vi "Error.vi"(8 "error in (no error)":errorcluster, 11 "Data":variant) -> (0 "error out":errorcluster)   [LabVIEW 2014, in "Testing UI 1.lvlib"]
doc: "This subVI enqueues the named action in to the communications queue along with the input data."
uses:
  Testing UI 1.lvlib
  Private Controls/Module Data.ctl
  Private Controls/Module Action.ctl
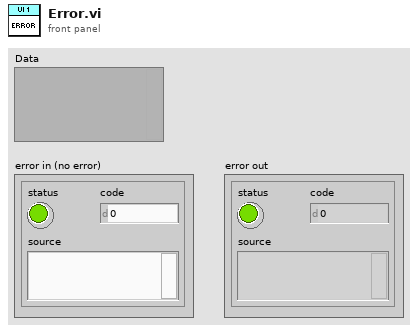
[diagram p1: front panel]
types:
  T1 = typedef "Testing UI 1.lvlib/Module Data.ctl" = cluster{"Data":variant, "Action":T2}
  T2 = typedef "Testing UI 1.lvlib/Module Action.ctl" = enum8{"Init", "Error", "Exit", "HideShow FP", "Send Control Vals", "New Message Line", "Update System Log", "Load APU Setup Data", "Update APU Name", "Set Testing Type", "Threshold ALERT", "Set Rapid OpenORClose", "Engine Start Val Change", "Fault Trip Run Updater", " ---------------UI 4 APIs ---------------", "UI 4 Engine Start Val Change", "UI 4 Fuel Pressure Reg Val Change", "U1 4 APU & ECU Control Val Change", "UI 4 Bleed Load Val Change", "UI4 Testing Controls Val Change", "UI4 Break Out Val Change", "UI4 Crash Log Val Change", "UI4 Log Data Val Change", "UI4 Sampes-Sec Val Change", "Update Run Count", "Config Interactive Ctrls"}
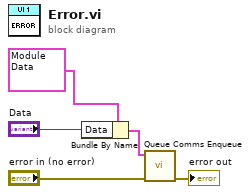
[diagram p0: block diagram]
diagram:
  n1 = Bundle By Name(cluster=T1 {"Data"=variant, "Action"=enum."Error"} ("element"), "Data"="Data") -> (w4:T1)
  n2 = call "Queue Comms Enqueue.vi"("error in (no error)"="error in (no error)", "element"=w4) -> ("error out"=→"error out":errorcluster)  [unwired: 9 in]
